vi "Initialize.vi"(7 "ChannelName":string="Setpoint.ch%d.SP", 8 "error in":errorcluster, 9 "Number of Channels":u32=1, 10 "Instance Name":string, 11 "Climate Chamber in":refnum<class "Climate Chamber.lvclass">) -> (0 "error out":errorcluster, 2 "Channel":T1[](array[typedef]), 3 "Climate Chamber out":refnum<class "Climate Chamber.lvclass">)   [LabVIEW 2023, in "Climate Chamber.lvclass"]
uses:
  Climate Chamber.lvclass
  Utilities/Channel.ctl
  Climate Chamber.lvclass/Climate Chamber.ctl
  Low Level Capabilities/OnOff/OnOff.lvclass
  Low Level Capabilities/Temperature/Temperature Setpoint/Temperature Setpoint.lvclass
  Low Level Capabilities/Temperature/Temperature Actual Value/Temperature Actual Value.lvclass
  Low Level Capabilities/Error/Error.lvclass
  Low Level Capabilities/Temperature/Temperature Gradient/Temperature Gradient.lvclass
  Low Level Capabilities/Temperature/Temperature Limit/Temperature Limit.lvclass
  Low Level Capabilities/Humidity/Humidity Setpoint/Humidity Setpoint.lvclass
  Low Level Capabilities/Humidity/Humidity Limit/Humidity Limit.lvclass
  Low Level Capabilities/Humidity/Humidity Gradient/Humidity Gradient.lvclass
  Low Level Capabilities/Humidity/Humidity Actual Value/Humidity Actual Value.lvclass
  Utilities/Utilities.lvlib
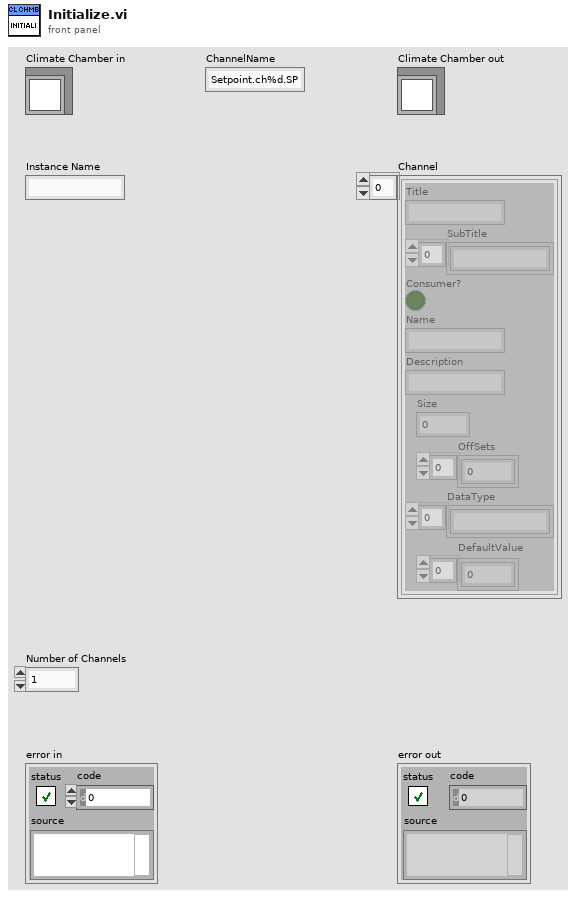
[diagram p1: front panel]
types:
  T1 = typedef "Utilities.lvlib/Channel.ctl" = cluster{"Title":string, "SubTitle":string[], "Consumer?":bool, "Name":string, "Description":string, "Size":i32, "OffSets":i32[], "DataType":string[], "DefaultValue":dbl[]}
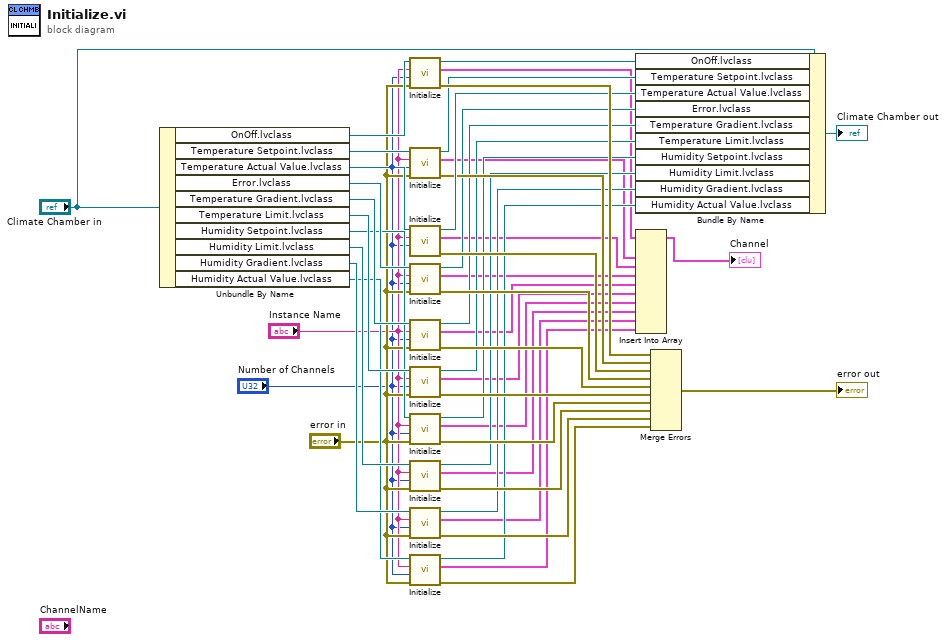
[diagram p0: block diagram]
diagram:
  n1 = Unbundle By Name("Climate Chamber in") -> ("OnOff.lvclass"=w44:refnum<class "OnOff.lvclass">, "Temperature Setpoint.lvclass"=w41:refnum<class "Temperature Setpoint.lvclass">, "Temperature Actual Value.lvclass"=w39:refnum<class "Temperature Actual Value.lvclass">, "Error.lvclass"=w35:refnum<class "Error.lvclass">, "Temperature Gradient.lvclass"=w32:refnum<class "Temperature Gradient.lvclass">, "Temperature Limit.lvclass"=w29:refnum<class "Temperature Limit.lvclass">, "Humidity Setpoint.lvclass"=w26:refnum<class "Humidity Setpoint.lvclass">, "Humidity Limit.lvclass"=w23:refnum<class "Humidity Limit.lvclass">, "Humidity Gradient.lvclass"=w20:refnum<class "Humidity Gradient.lvclass">, "Humidity Actual Value.lvclass"=w17:refnum<class "Humidity Actual Value.lvclass">)
  n2 = call-dynamic "Initialize.vi"("error in"="error in", "Number of Channels"="Number of Channels", "Instance Name"="Instance Name", "OnOff in"=w44) -> ("error out"=w42:errorcluster, "Channel"=w11:T1[], "OnOff out"=w43:refnum<class "OnOff.lvclass">)  [unwired: 5 in]
  n3 = call-dynamic "Initialize.vi"("error in"="error in", "Number of Channels"="Number of Channels", "Instance Name"="Instance Name", "Temperature Setpoint in"=w41) -> ("error out"=w37:errorcluster, "Channel"=w10:T1[], "Temperature Setpoint out"=w40:refnum<class "Temperature Setpoint.lvclass">)  [unwired: 5 in]
  n4 = call-dynamic "Initialize.vi"("Number of Channels"="Number of Channels", "Instance Name"="Instance Name", "Temperature Actual Value in"=w39) -> ("error out"=w36:errorcluster, "Channel"=w9:T1[], "Temperature Actual Value out"=w38:refnum<class "Temperature Actual Value.lvclass">)  [unwired: 6 in]
  n5 = call-dynamic "Initialize.vi"("error in"="error in", "Number of Channels"="Number of Channels", "Instance Name"="Instance Name", "Error in"=w35) -> ("error out"=w33:errorcluster, "Channel"=w8:T1[], "Error out"=w34:refnum<class "Error.lvclass">)  [unwired: 5 in]
  n6 = call-dynamic "Initialize.vi"("error in"="error in", "Number of Channels"="Number of Channels", "Instance Name"="Instance Name", "Temperature Gradient in"=w32) -> ("error out"=w30:errorcluster, "Channel"=w7:T1[], "Temperature Gradient out"=w31:refnum<class "Temperature Gradient.lvclass">)  [unwired: 5 in]
  n7 = call-dynamic "Initialize.vi"("error in"="error in", "Number of Channels"="Number of Channels", "Instance Name"="Instance Name", "Temperature Limit in"=w29) -> ("error out"=w27:errorcluster, "Channel"=w6:T1[], "Temperature Limit out"=w28:refnum<class "Temperature Limit.lvclass">)  [unwired: 5 in]
  n8 = call-dynamic "Initialize.vi"("error in"="error in", "Number of Channels"="Number of Channels", "Instance Name"="Instance Name", "Humidity Setpoint in"=w26) -> ("error out"=w24:errorcluster, "Channel"=w5:T1[], "Humidity Setpoint out"=w25:refnum<class "Humidity Setpoint.lvclass">)  [unwired: 5 in]
  n9 = call-dynamic "Initialize.vi"("error in"="error in", "Number of Channels"="Number of Channels", "Instance Name"="Instance Name", "Humidity Limit in"=w23) -> ("error out"=w21:errorcluster, "Channel"=w4:T1[], "Humidity Limit out"=w22:refnum<class "Humidity Limit.lvclass">)  [unwired: 5 in]
  n10 = call-dynamic "Initialize.vi"("error in"="error in", "Number of Channels"="Number of Channels", "Instance Name"="Instance Name", "Humidity Gradient in"=w20) -> ("error out"=w18:errorcluster, "Channel"=w3:T1[], "Humidity Gradient out"=w19:refnum<class "Humidity Gradient.lvclass">)  [unwired: 5 in]
  n11 = call-dynamic "Initialize.vi"("error in"="error in", "Number of Channels"="Number of Channels", "Instance Name"="Instance Name", "Humidity Actual Value in"=w17) -> ("error out"=w15:errorcluster, "Channel"=w2:T1[], "Humidity Actual Value out"=w16:refnum<class "Humidity Actual Value.lvclass">)  [unwired: 5 in]
  n12 = Bundle By Name(cluster="Climate Chamber in", "OnOff.lvclass"=w43, "Temperature Setpoint.lvclass"=w40, "Temperature Actual Value.lvclass"=w38, "Error.lvclass"=w34, "Temperature Gradient.lvclass"=w31, "Temperature Limit.lvclass"=w28, "Humidity Setpoint.lvclass"=w25, "Humidity Limit.lvclass"=w22, "Humidity Gradient.lvclass"=w19, "Humidity Actual Value.lvclass"=w16) -> (→"Climate Chamber out":refnum<class "Climate Chamber.lvclass">)
  n13 = Insert Into Array(array=w11, new element #1=w10, new element #2=w9, new element #3=w8, new element #4=w7, new element #5=w6, new element #6=w5, new element #7=w4, new element #8=w3, new element #9=w2) -> (→"Channel":T1[])  [unwired: 1 in]
  n14 = Merge Errors(w42, w37, w36, w33, w30, w27, w24, w21, w18, w15) -> (→"error out":errorcluster)
